vi "End Turn.vi"(6 "Error":errorcluster, 7 "Actor":refnum<class "Actor Layer.lvclass">, 11 "Actor":T1) -> (2 "Teardown":bool, 3 "Actor":T1, 4 "Error":errorcluster, 5 "Actor":refnum<class "Actor Layer.lvclass">)   [LabVIEW 2020, in "jettl.lvlib"]
uses:
  jettl.lvlib
  Lifecycle.ctl
  Actor Layer/Actor Layer.lvclass
  Msg/Msg.lvclass
  Msg.ctl
  Post Setup.ctl
  Pre Setup.ctl
  Msg Set.ctl
  Actor Attribs.ctl
  Children.ctl
  Actor.ctl
  Origin.ctl
  Msg Attribs.ctl
  Layer Type.ctl
  Layer Attribs.ctl
  Layer Map.ctl
  Implemented Map.ctl
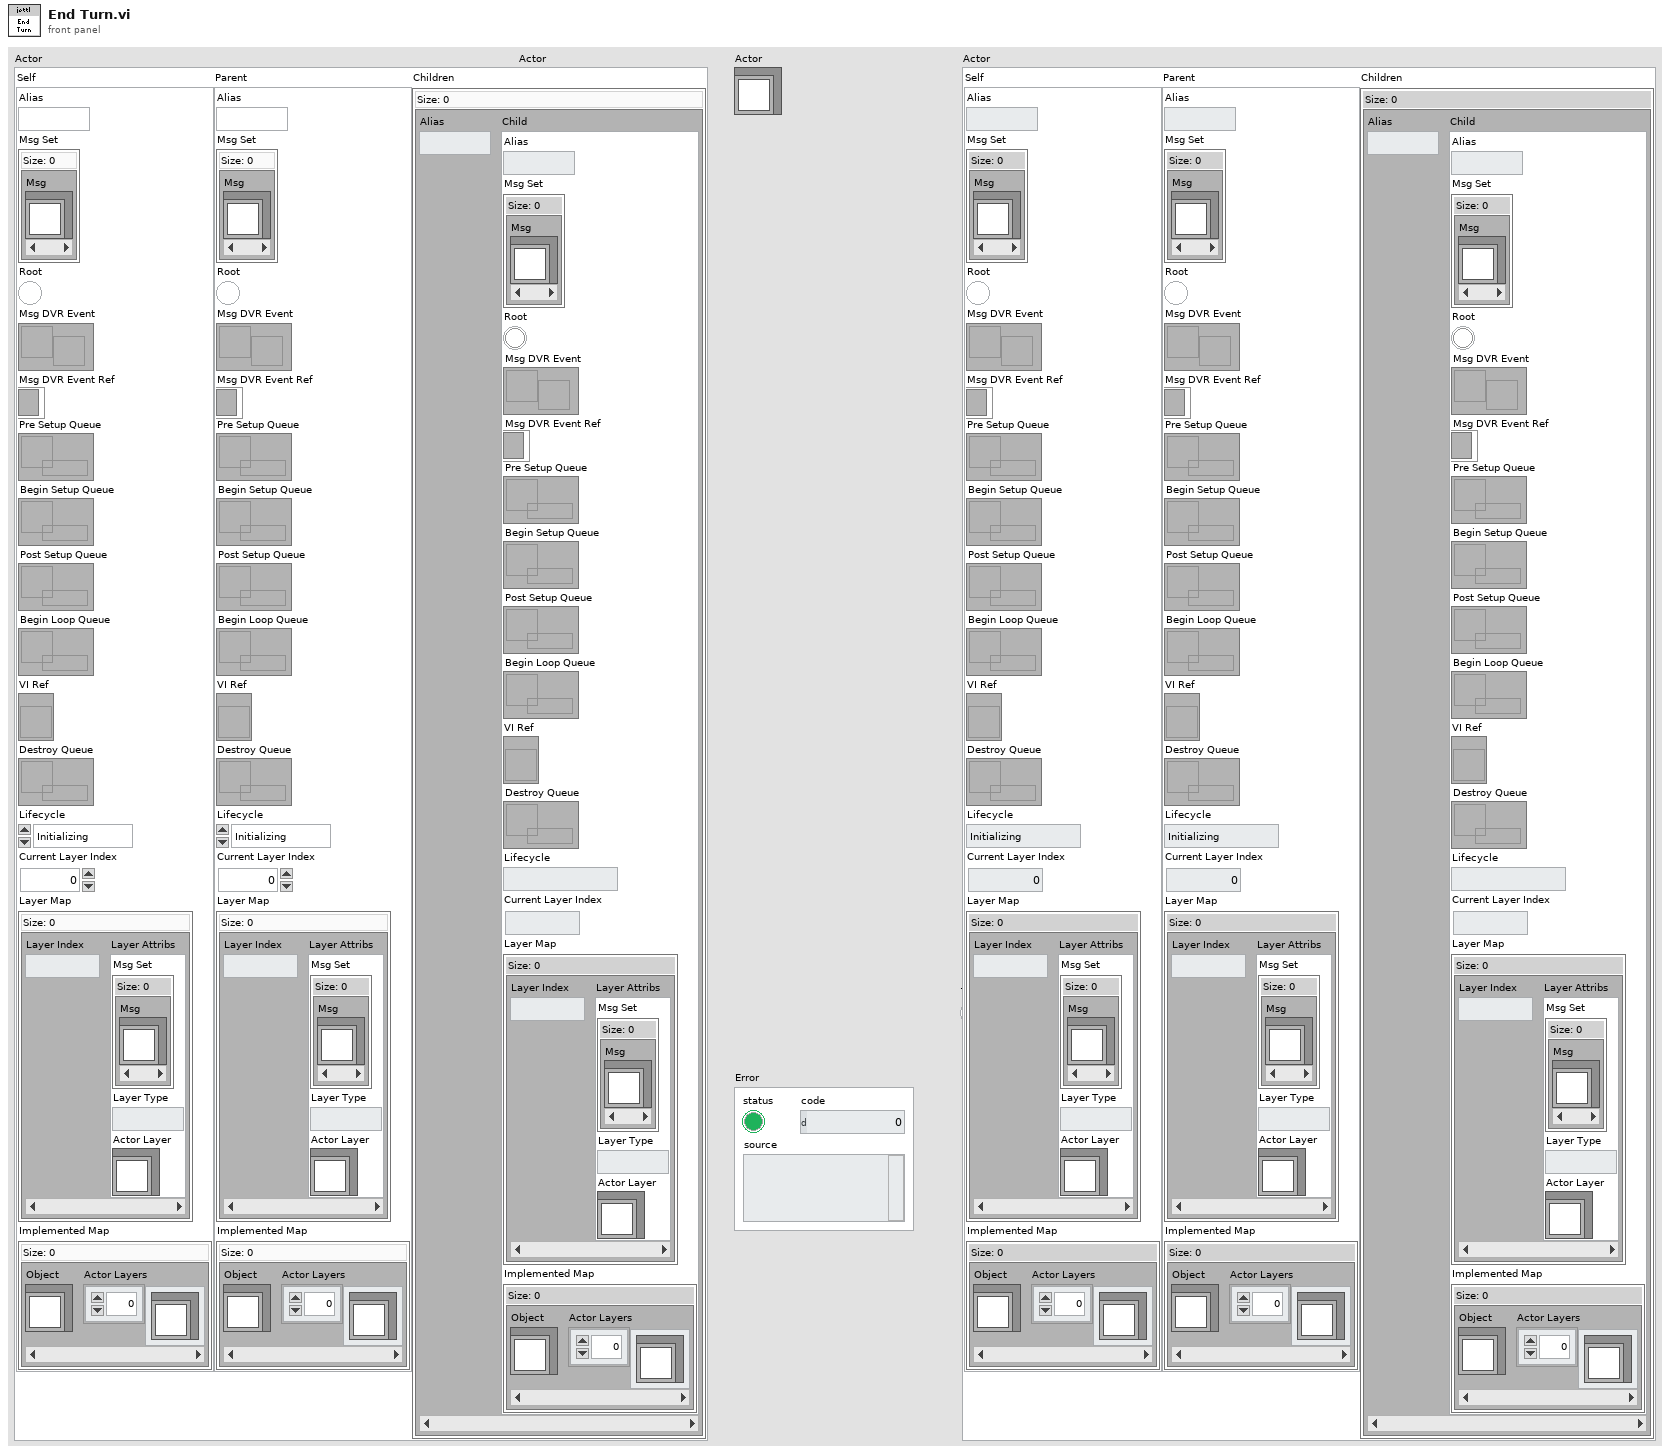
[diagram p1: front panel]
types:
  T1 = typedef "jettl.lvlib/Actor.ctl" = cluster{"Self":T2, "Parent":T2, "Children":T9}
  T2 = typedef "jettl.lvlib/Actor Attribs.ctl" = cluster{"Alias":string, "Msg Set":T3, "Root":bool, "Msg DVR Event":refnum<user-event>, "Msg DVR Event Ref":refnum<event-registration>, "Pre Setup Queue":refnum<queue>, "Begin Setup Queue":refnum<queue>, "Post Setup Queue":refnum<queue>, "Begin Loop Queue":refnum<queue>, "VI Ref":refnum<vi>, "Destroy Queue":refnum<queue>, "Lifecycle":T4, "Current Layer Index":i32, "Layer Map":T5, "Implemented Map":T8}
  T3 = typedef "jettl.lvlib/Msg Set.ctl" = set{refnum<class "Msg.lvclass">}
  T4 = typedef "jettl.lvlib/Lifecycle.ctl" = enum16{"Initializing", "Setting Up", "Starting", "Running", "Stopping", "Tearing Down", "Terminated"}
  T5 = typedef "jettl.lvlib/Layer Map.ctl" = map{i32, T6}
  T6 = typedef "jettl.lvlib/Layer Attribs.ctl" = cluster{"Msg Set":T3, "Layer Type":T7, "Actor Layer":refnum<class "Actor Layer.lvclass">}
  T7 = typedef "jettl.lvlib/Layer Type.ctl" = enum16{"Base", "InnerGlobal", "InnerLocal", "Outer"}
  T8 = typedef "jettl.lvlib/Implemented Map.ctl" = map{refnum<class>, refnum<class "Actor Layer.lvclass">[]}
  T9 = typedef "jettl.lvlib/Children.ctl" = map{string, T2}
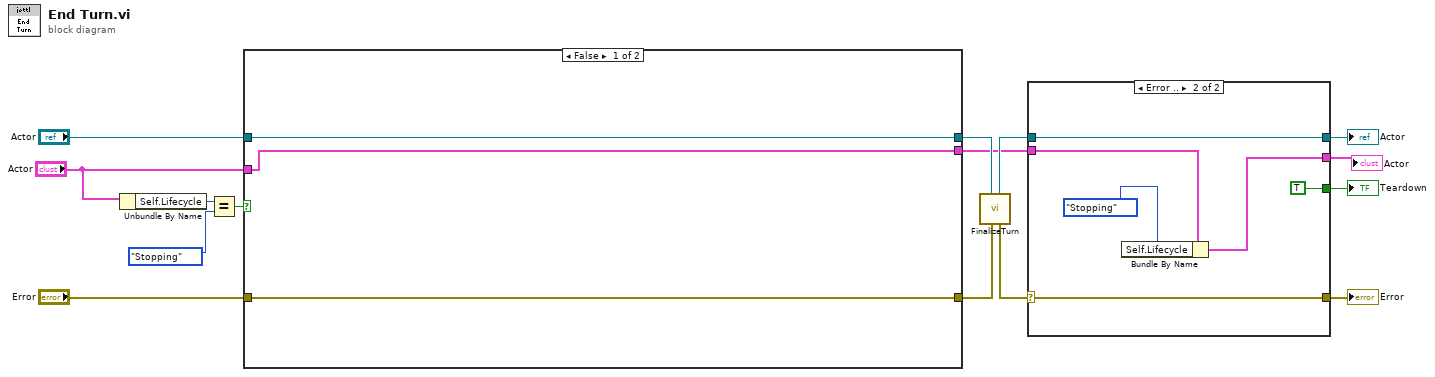
[diagram p0: block diagram]
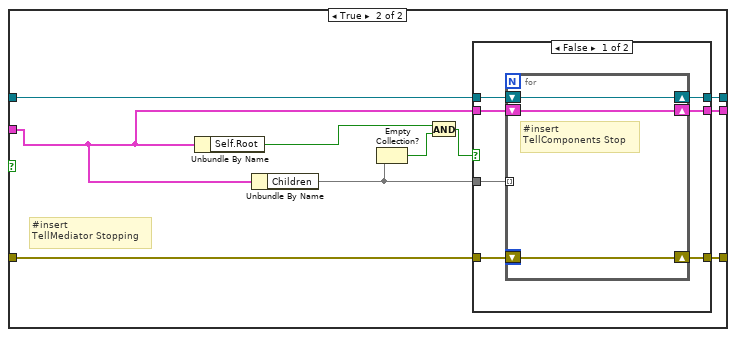
[diagram p2: hidden frame]
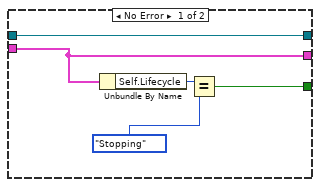
[diagram p4: hidden frame]
diagram:
  n1 = Unbundle By Name("Actor") -> ("Self.Lifecycle"=w12:T4)
  n2 = Equal?(x=w12, y=Lifecycle."Stopping") -> (x = y?=w14:bool)
  n3 = case shown="False" w14 {
    tunnel: "Error" -> [w18 w27]
    tunnel: [w18 w28] -> w9
    tunnel: [w17 w25] -> w10
    tunnel: "Actor" -> [w17 w24]
    tunnel: "Actor" -> [w16 w20]
    tunnel: [w16 w19] -> w2
    frame False {
    }
    frame True {
      # "#insert\nTellMediator Stopping"
      n4 = Unbundle By Name(w20) -> ("Self.Root"=w21:bool)
      n5 = Unbundle By Name(w20) -> ("Children"=w26:T9)
      n6 = Empty Collection?(1:w26) -> (0:w23:bool)
      n7 = And(x=w21, y=w23) -> (x .and. y?=w22:bool)
      n8 = case shown="False" w22 {
        tunnel: w27 -> [w35 w40]
        tunnel: [w34 w40] -> w28
        tunnel: w24 -> [w33 w41]
        tunnel: [w32 w41] -> w25
        tunnel: w26 -> [w31 _]
        tunnel: w20 -> [w30 w39]
        tunnel: [w29 w39] -> w19
        frame False {
          n9 = for {
            tunnel: w31 -> [_] mode=indexing
            shift-right: [w37] -> w34
            shift-left: w35 -> [w37]
            shift-right: [w38] -> w32
            shift-left: w33 -> [w38]
            shift-right: [w36] -> w29
            shift-left: w30 -> [w36]
            # "#insert\nTellComponents Stop"
          }
        }
        frame True {
        }
      }
    }
  }
  n10 = call-dynamic "FinalizeTurn.vi"("Error"=w9, "Actor"=w10) -> ("Error"=w8:errorcluster, "Actor"=w7:refnum<class "Actor Layer.lvclass">)  [unwired: 7 in, 1 out]
  n11 = case shown="Error .." w8 {
    selector: w8 -> [_ w52]
    tunnel: [_ w52] -> w15
    tunnel: w7 -> [w45 w47]
    tunnel: [w45 w47] -> w6
    tunnel: [w44 TRUE] -> w5
    tunnel: w2 -> [w42 w49]
    tunnel: [w42 w50] -> w1
    frame No Error {
      n12 = Unbundle By Name(w42) -> ("Self.Lifecycle"=w46:T4)
      n13 = Equal?(x=w46, y=Lifecycle."Stopping") -> (x = y?=w44:bool)
    }
    frame Error {
      n14 = Bundle By Name(cluster=w49, "Self.Lifecycle"=Lifecycle."Stopping" ("Lifecycle")) -> (w50:T1)
    }
  }
  "Actor" <- w6
  "Teardown" <- w5
  "Error" <- w15
  "Actor" <- w1
